vi "MSSQL_Update.vi"(0 "connection reference":T1, 1 "表名":string, 2 "修改条件":string, 3 "异常输入":errorcluster, 4 "列名数组":string[](array[string]), 5 "值数组":string[](array[string])) -> (6 "connection reference 2":T1, 7 "操作结果":bool, 9 "异常输出":errorcluster)   [LabVIEW 2018]
uses:
  <vilib>/addons/database/Connection.llb/Conn ObjectReference.ctl
  <vilib>/addons/database/Connection.llb/Conn Execute.vi
  <vilib>/addons/database/Recordset.llb/Rec Destroy - Connection.vi
  <vilib>/addons/database/NI_Database_API.lvlib
panel:
  # "update操作\nupdate tbl_name set 列1 = ‘值1’，列2 = ‘值2’ where 列1 = ‘1’"
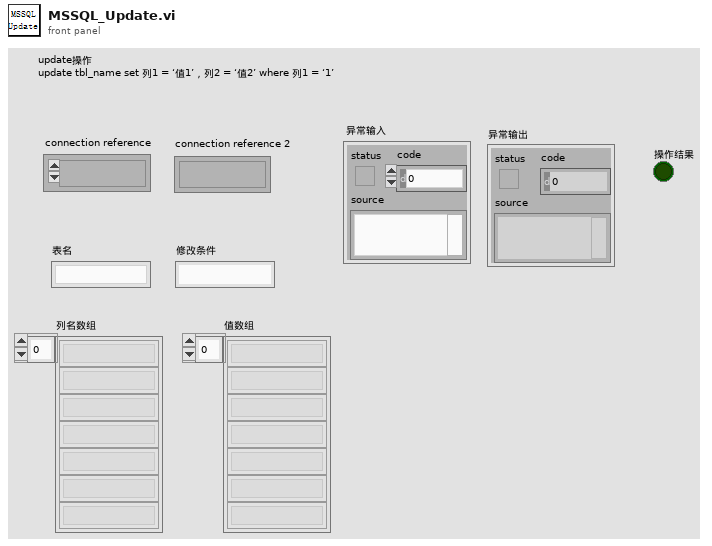
[diagram p1: front panel]
types:
  T1 = typedef "NI_Database_API.lvlib/Conn ObjectReference.ctl" = refnum<k1>
  T2 = typedef "NI_Database_API.lvlib/Rec ObjectReference.ctl" = refnum<k1>
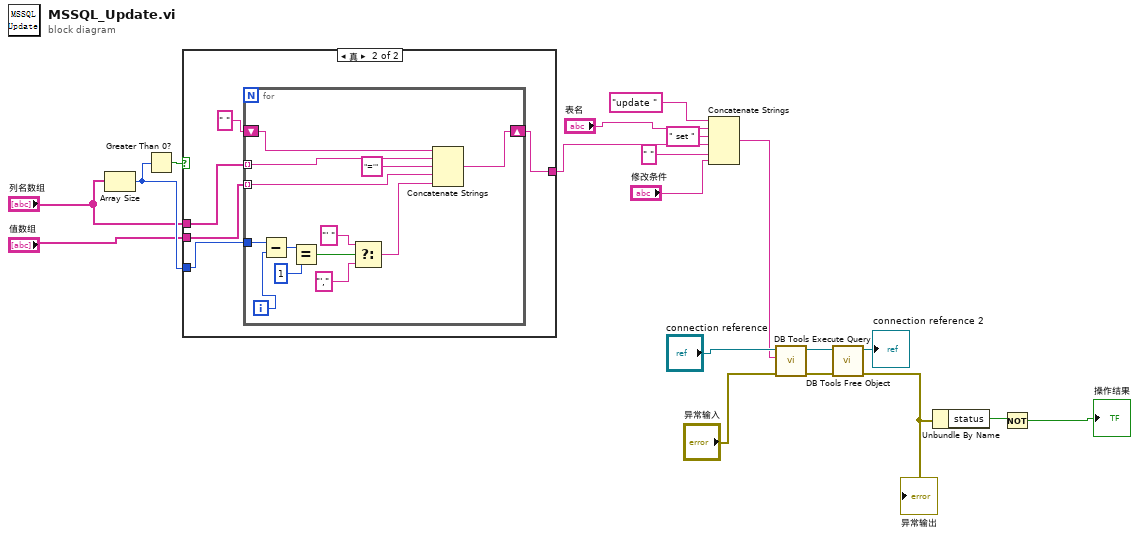
[diagram p0: block diagram]
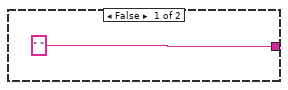
[diagram p2: hidden frame]
diagram:
  n1 = Array Size(array="列名数组") -> (size(s)=w17:i32)
  n2 = Greater Than 0?(x=w17) -> (x > 0?=w18:bool)
  n3 = case shown="真" w18 {
    tunnel: [" " w22] -> w8
    tunnel: w17 -> [_ w25]
    tunnel: "列名数组" -> [_ w24]
    tunnel: "值数组" -> [_ w21]
    frame False {
    }
    frame True {
      n4 = for {
        tunnel: w24 -> [w37] mode=indexing
        shift-right: [w36] -> w22
        shift-left: " " -> [w38]
        tunnel: w25 -> [w29]
        tunnel: w21 -> [w27] mode=indexing
        i -> [w35]
        n5 = Subtract(x=w29, y=w35) -> (x-y=w34:i32)
        n6 = Equal?(x=w34, y=1) -> (x = y?=w32:bool)
        n7 = Select(t="' " ("字符串"), s=w32, f="',") -> (s? t:f=w26:string)
        n8 = Concatenate Strings(w38, w37, "='" ("字符串"), w27, w26) -> (w36:string)
      }
    }
  }
  n9 = Concatenate Strings("update ", "表名", " set " ("字符串"), w8, " " ("字符串"), "修改条件") -> (w15:string)
  n10 = call-poly <vilib>:"DB Tools Execute Query.vi"("error in (no error)"="异常输入", "SQL query"=w15, "connection reference"="connection reference") -> ("error out"=w13:errorcluster, "recordset reference"=w14:T2)  [unwired: 5 in]
  n11 = call-poly <vilib>:"DB Tools Free Object.vi"("error in (no error)"=w13, "recordset reference"=w14) -> ("error out"=w10:errorcluster, "connection reference"=→"connection reference 2":T1)  [unwired: 8 in]
  "异常输出" <- w10
  n12 = Unbundle By Name(w10) -> ("status"=w2:bool)
  n13 = Not(x=w2) -> (.not. x?=→"操作结果":bool)
